vi "Clear Private Data Cluster.vi"(8 "error in (no error)":errorcluster, 11 "LVClassLibrary in":refnum<vi>) -> (0 "error out":errorcluster, 3 "LVClassLibrary out":refnum<vi>)   [LabVIEW 2019, in "gRPC Template Creation Utility.lvlib"]
uses:
  gRPC Template Creation Utility.lvlib
  <vilib>/Utility/traverseref.llb/VI Scripting - Traverse.lvlib
  <vilib>/Utility/traverseref.llb/TRef TravTarget.ctl
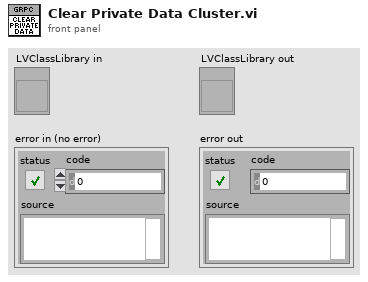
[diagram p1: front panel]
types:
  T1 = typedef "TRef TravTarget.ctl" = enum16{"FP", "BD", "Other"}
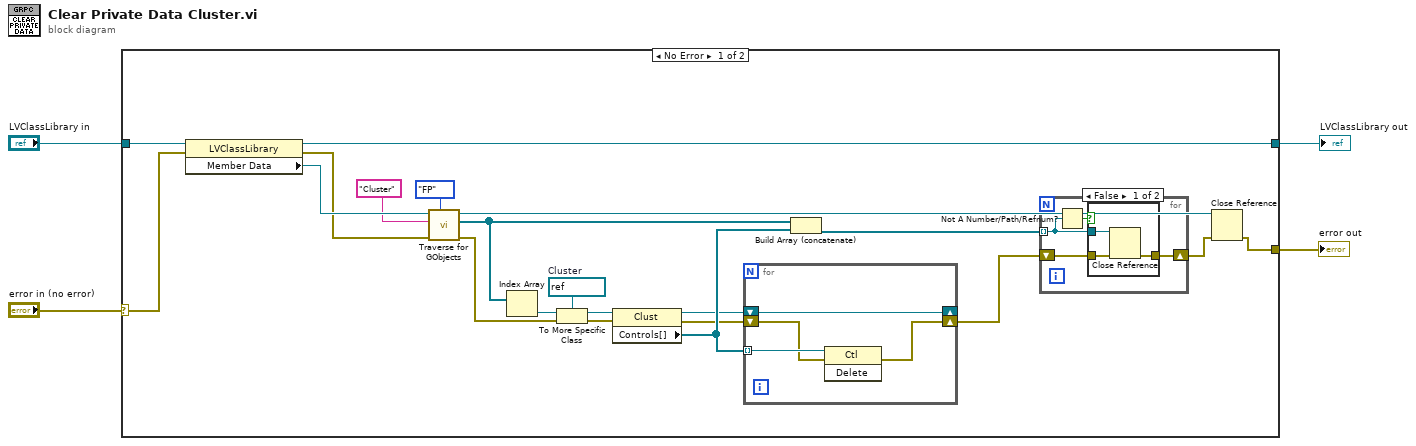
[diagram p0: block diagram]
diagram:
  n1 = case shown="No Error" "error in (no error)" {
    selector: "error in (no error)" -> [w8 w38]
    tunnel: [w25 w39] -> w4
    tunnel: "LVClassLibrary in" -> [w24 w39]
    tunnel: [w9 w38] -> w2
    frame No Error {
      w17 = refnum<vi> refnum  # Cluster
      n2 = property class="LVClassLibrary"(reference=w24, error in=w8) -> (reference out=w25:refnum<vi>, error out=w14:errorcluster, "Member Data"=w19:refnum<vi>)
      n3 = call <vilib>:"Traverse for GObjects.vi"("Traverse Target"=TRef_TravTarget."FP", "error in (no error)"=w14, "Class Name"="Cluster" ("name/order"), "VI Refnum"=w19) -> ("error out"=w18:errorcluster, "References"=w20:refnum<vi>[], "dup VI Refnum"=w10:refnum<vi>)  [unwired: 4 in, 1 out]
      n4 = Index Array(array=w20) -> (element=w15:refnum<vi>)  [unwired: 1 in]
      n5 = To More Specific Class(target class=w17, reference=w15, error in=w18) -> (specific class reference=w16:refnum<vi>, error out=w21:errorcluster)
      n6 = property class="Clust"(reference=w16, error in=w21) -> (reference out=w22:refnum<vi>, error out=w11:errorcluster, "Controls[]"=w23:refnum<vi>[])
      n7 = for {
        shift-right: [w37] -> _
        shift-left: w22 -> [w37]
        shift-right: [w34] -> w6
        shift-left: w11 -> [w35]
        tunnel: w23 -> [w36] mode=indexing
        n8 = invoke class="Ctl" method="Delete"(reference=w36, error in=w35) -> (error out=w34:errorcluster)  [unwired: 1 in, 2 out]
      }
      n9 = Build Array (concatenate)(w20, w23) -> (w7:refnum<vi>[])
      n10 = for {
        tunnel: w7 -> [w28] mode=indexing
        shift-right: [w26] -> w5
        shift-left: w6 -> [w27]
        n11 = Not A Number/Path/Refnum?(number/path/refnum=w28) -> (NaN/Path/Refnum?=w29:bool)
        n12 = case shown="False" w29 {
          tunnel: w28 -> [w32 _]
          tunnel: w27 -> [w31 w33]
          tunnel: [w30 w33] -> w26
          frame False {
            n13 = Close Reference(reference=w32, error in (no error)=w31) -> (error out=w30:errorcluster)
          }
          frame True {
          }
        }
      }
      n14 = Close Reference(reference=w10, error in (no error)=w5) -> (error out=w9:errorcluster)
    }
    frame Error {
    }
  }
  "LVClassLibrary out" <- w4
  "error out" <- w2
